vi "Item_OnCommand.vi"(10 "Command ID":string, 11 "Object":T1) -> ()   [LabVIEW 2020, in "Project Provider.lvlib"]
uses:
  Project Provider.lvlib
  <resource>/Framework/Providers/API/ItemRef.ctl
panel:
  out "error out":errorcluster
  in  "error in":errorcluster
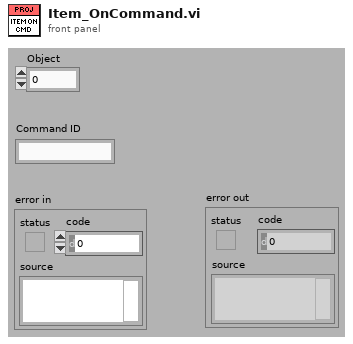
[diagram p1: front panel]
types:
  T1 = typedef "ItemRef.ctl" = u64
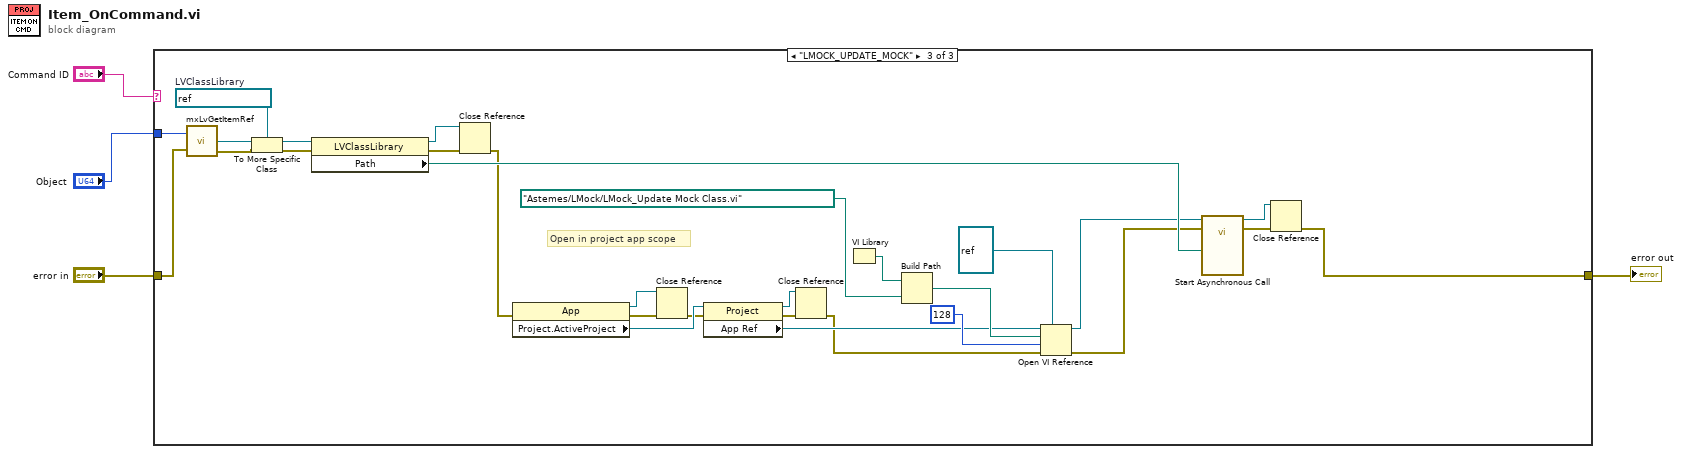
[diagram p0: block diagram]
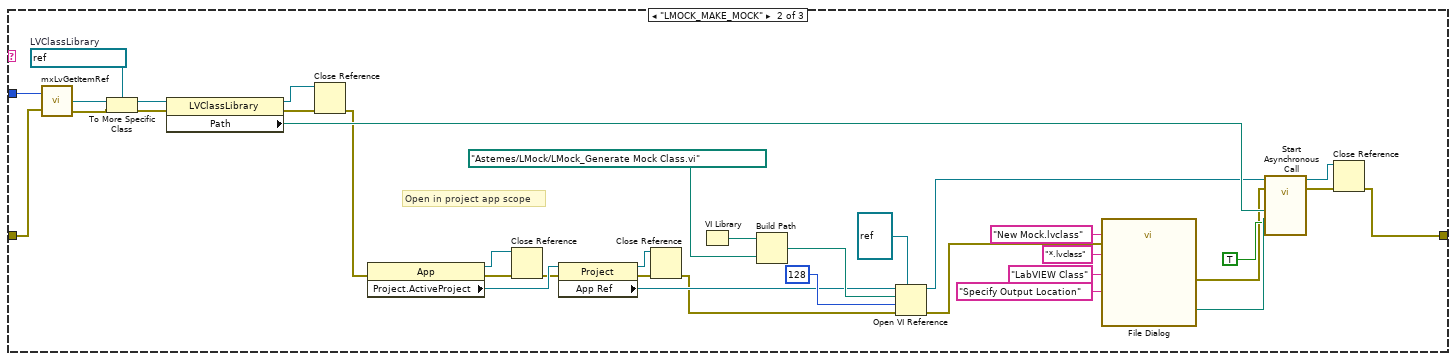
[diagram p3: hidden frame]
diagram:
  n1 = case shown="\"LMOCK_UPDATE_MOCK\"" "Command ID" {
    tunnel: "error in" -> [w5 w40 w69]
    tunnel: [w5 w15 w45] -> w2
    tunnel: "Object" -> [_ w41 w70]
    frame Default {
    }
    frame "LMOCK_MAKE_MOCK" {
      w37 = refnum<vi> refnum  # LVClassLibrary
      # "Open in project app scope"
      n2 = call <resource>:"mxLvGetItemRef.vi"("Item"=w41, "error in"=w40) -> ("Item Refnum"=w39:refnum<vi>, "error out"=w30:errorcluster)  [unwired: 1 out]
      n3 = To More Specific Class(target class=w37, reference=w39, error in=w30) -> (specific class reference=w38:refnum<vi>, error out=w36:errorcluster)
      n4 = property class="LVClassLibrary"(reference=w38, error in=w36) -> (reference out=w34:refnum<vi>, error out=w35:errorcluster, "Path"=w32:path)
      n5 = Close Reference(reference=w34, error in (no error)=w35) -> (error out=w26:errorcluster)
      n6 = property class="App"(error in=w26) -> (reference out=w16:refnum<vi>, error out=w18:errorcluster, "Project.ActiveProject"=w23:refnum<vi>)  [unwired: 1 in]
      n7 = Close Reference(reference=w16, error in (no error)=w18) -> (error out=w17:errorcluster)
      n8 = property class="Project"(reference=w23, error in=w17) -> (reference out=w22:refnum<vi>, error out=w20:errorcluster, "App Ref"=w21:refnum<vi>)
      n9 = Close Reference(reference=w22, error in (no error)=w20) -> (error out=w19:errorcluster)
      n10 = VI Library() -> (path=w24:path)
      n11 = Build Path(base path=w24, name or relative path=path "Astemes/LMock/LMock_Generate Mock Class.vi" ("Relative Path from 1 to 2")) -> (appended path=w29:path)
      n12 = Open VI Reference(type specifier VI Refnum (for type only)=refnum<vi> refnum, application reference (local)=w21, vi path=w29, options=128, error in (no error)=w19) -> (vi reference=w28:refnum<vi>, error out=w8:errorcluster)  [unwired: 1 in]
      n13 = call "File Dialog"("prompt"="Specify Output Location", "default name"="New Mock.lvclass", "error in"=w8, "pattern (all files)"="*.lvclass", "pattern label"="LabVIEW Class") -> ("selected path"=w11:path, "error out"=w7:errorcluster)  [unwired: 7 in, 2 out]
      n14 = call-by-ref "Start Asynchronous Call"(reference=w28, error in=w7, "Add to lvproj?"=TRUE, "Destination Class Path"=w11, "Source Class Path"=w32) -> (reference out=w31:refnum<vi>, error out=w33:errorcluster)  [unwired: 7 in, 2 out]
      n15 = Close Reference(reference=w31, error in (no error)=w33) -> (error out=w15:errorcluster)
    }
    frame "LMOCK_UPDATE_MOCK" {
      w66 = refnum<vi> refnum  # LVClassLibrary
      # "Open in project app scope"
      n16 = call <resource>:"mxLvGetItemRef.vi"("Item"=w70, "error in"=w69) -> ("Item Refnum"=w68:refnum<vi>, "error out"=w59:errorcluster)  [unwired: 1 out]
      n17 = To More Specific Class(target class=w66, reference=w68, error in=w59) -> (specific class reference=w67:refnum<vi>, error out=w65:errorcluster)
      n18 = property class="LVClassLibrary"(reference=w67, error in=w65) -> (reference out=w63:refnum<vi>, error out=w64:errorcluster, "Path"=w61:path)
      n19 = Close Reference(reference=w63, error in (no error)=w64) -> (error out=w55:errorcluster)
      n20 = property class="App"(error in=w55) -> (reference out=w46:refnum<vi>, error out=w48:errorcluster, "Project.ActiveProject"=w53:refnum<vi>)  [unwired: 1 in]
      n21 = Close Reference(reference=w46, error in (no error)=w48) -> (error out=w47:errorcluster)
      n22 = property class="Project"(reference=w53, error in=w47) -> (reference out=w52:refnum<vi>, error out=w50:errorcluster, "App Ref"=w51:refnum<vi>)
      n23 = Close Reference(reference=w52, error in (no error)=w50) -> (error out=w49:errorcluster)
      n24 = VI Library() -> (path=w42:path)
      n25 = Build Path(base path=w42, name or relative path=path "Astemes/LMock/LMock_Update Mock Class.vi" ("Relative Path from 1 to 2")) -> (appended path=w58:path)
      n26 = Open VI Reference(type specifier VI Refnum (for type only)=refnum<vi> refnum, application reference (local)=w51, vi path=w58, options=128, error in (no error)=w49) -> (vi reference=w57:refnum<vi>, error out=w44:errorcluster)  [unwired: 1 in]
      n27 = call-by-ref "Start Asynchronous Call"(reference=w57, error in=w44, "Source Class Path"=w61) -> (reference out=w60:refnum<vi>, error out=w62:errorcluster)  [unwired: 10 in, 1 out]
      n28 = Close Reference(reference=w60, error in (no error)=w62) -> (error out=w45:errorcluster)
    }
  }
  "error out" <- w2
